vi "Add Marker.vi"(0 ".NET Refnum In":refnum<k24>, 1 "Inputs":T3, 3 "ToolTip Text":string="Base", 4 "Marker Tooltip":i32(ring) items=["On Mouse Over", "Never", "Always"], 5 "Marker Type":T1(ring)=enum."arrow") -> (8 "arrOverlayRefs":refnum<k24>[](array[refnum]), 12 ".NET Refnum Out":refnum<k24>, 14 "RefPointsColl - Out":refnum<k24>, 15 "arrPtKyOrId":string[](array[string]), 16 "arrLat|LngActv":dbl[][](array[numeric]), 17 "MarkersCount":i32, 18 "QFNs":cluster{"FN":T4, "Data":variant}[](array[cluster]))   [LabVIEW 2021, in "NMEA_GPS Ublox M8N.lvlib"]
uses:
  NMEA_GPS Ublox M8N.lvlib
  D:/My Projects/Ava Sanjesh Project/VI/GPS uBlox M8N Read/With GMap1.7.0/Data/GMap.NET.WindowsForms.dll
  Data/GMap.NET.WindowsForms.dll
  ctlSeqFNs.ctl
  ctlInput4PtsColl.ctl
  D:/My Projects/Ava Sanjesh Project/VI/GPS uBlox M8N Read/With GMap1.7.0/Data/GMap.NET.Core.dll
  Data/GMap.NET.Core.dll
  System.Drawing
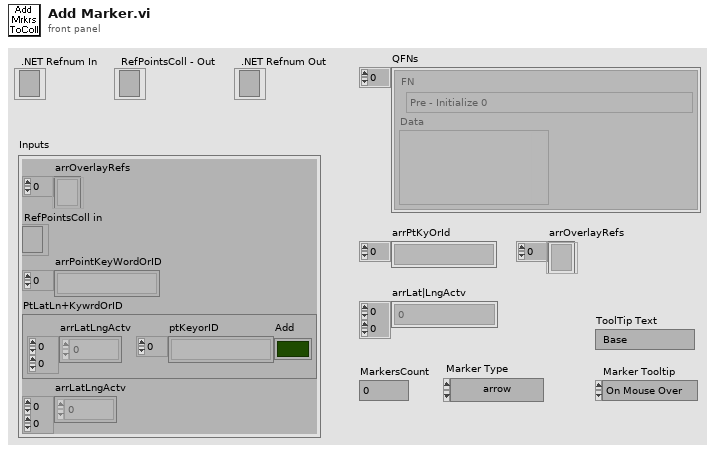
[diagram p1: front panel]
types:
  T1 = enum16{"none", "arrow", "blue", "blue_small", "blue_dot", "blue_pushpin", "brown_small", "gray_small", "green", "green_small", "green_dot", "green_pushpin", "green_big_go", "yellow", "yellow_small", "yellow_dot", "yellow_big_pause", "yellow_pushpin", "lightblue", "lightblue_dot", "lightblue_pushpin", "orange", "orange_small", "orange_dot", "pink", "pink_dot", "pink_pushpin", "purple", "purple_small", "purple_dot", "purple_pushpin", "red", "red_small", "red_dot", "red_pushpin", "red_big_stop", "black_small", "white_small"}
  T2 = typedef "NMEA_GPS Ublox M8N.lvlib/ctlInput4PtsColl.ctl" = cluster{"arrLatLngActv":dbl[][], "ptKeyorID":string[], "Add":bool}
  T3 = cluster{"arrOverlayRefs":refnum<k24>[], "RefPointsColl in":refnum<k24>, "arrPointKeyWordOrID":string[], "PtLatLn+KywrdOrID":T2, "arrLatLngActv":dbl[][]}
  T4 = typedef "NMEA_GPS Ublox M8N.lvlib/ctlSeqFNs.ctl" = enum16{"Pre - Initialize 0", "Pre - Initialize 1", "Pre - Initialize 2", "Pre - Initialize 3", "Idle", "Set Provider", "Set Scale", "Add Overlay", "Points - Create List (Container)", "Map - Marker Add Or Rmv", "Map - Markers Autofit", "Map - Markers Clear", "Error", "Exit"}
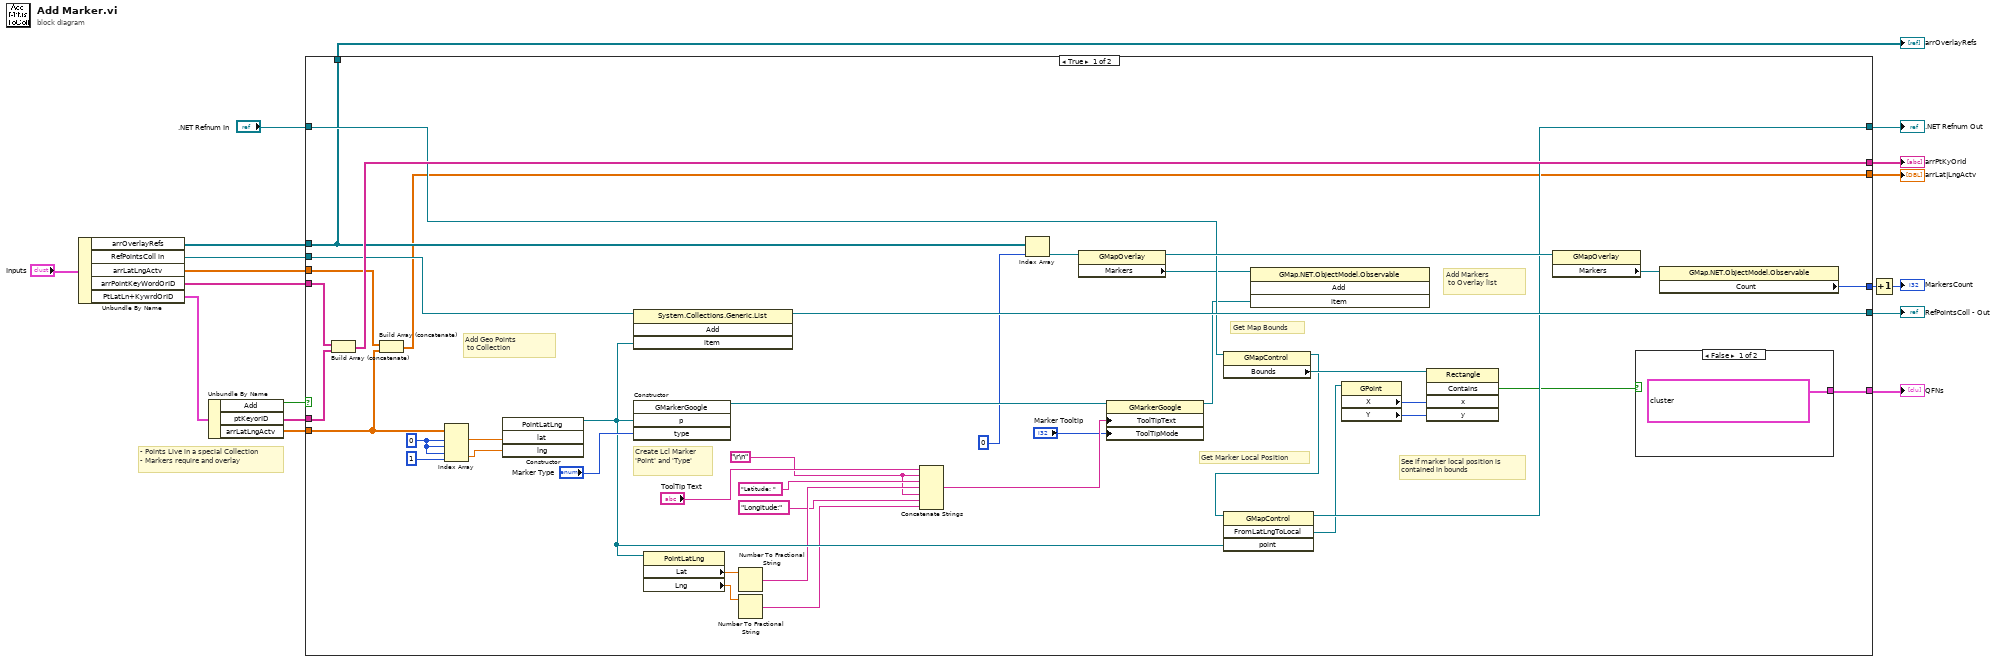
[diagram p0: block diagram]
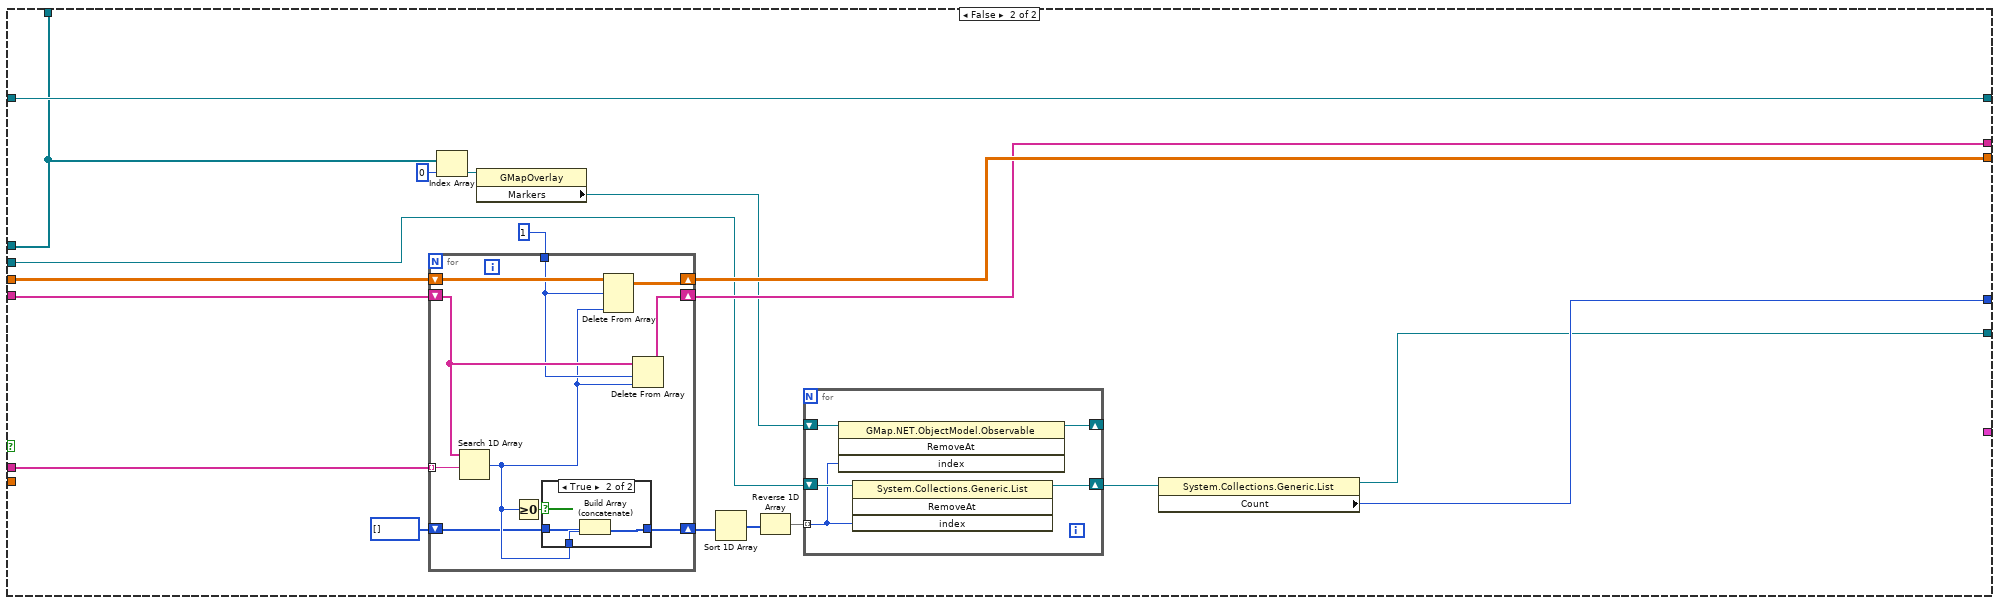
[diagram p3: hidden frame]
diagram:
  # "- Points Live in a special Collection\n- Markers require and overlay"
  n1 = Unbundle By Name("Inputs") -> ("arrOverlayRefs"=w10:refnum<k24>[], "RefPointsColl in"=w9:refnum<k24>, "arrLatLngActv"=w8:dbl[][], "arrPointKeyWordOrID"=w6:string[], "PtLatLn+KywrdOrID"=w7:T2)
  n2 = Unbundle By Name(w7) -> ("Add"=w2:bool, "ptKeyorID"=w12:string[], "arrLatLngActv"=w13:dbl[][])
  n3 = case shown="True" w2 {
    tunnel: [w60 _] -> w18
    tunnel: [w59 w74] -> w17
    tunnel: [w55 w75] -> w16
    tunnel: [w20 w76] -> w15
    tunnel: [w54 w65] -> w14
    tunnel: w13 -> [w53 _]
    tunnel: w12 -> [w52 w79]
    tunnel: w10 -> [w47 w63]
    tunnel: w9 -> [w51 w67]
    tunnel: w8 -> [w50 w78]
    tunnel: w6 -> [w49 w80]
    tunnel: ".NET Refnum In" -> [w48 w64]
    tunnel: [w46 w64] -> w3
    tunnel: [w47 w63] -> w4
    frame True {
      w25 = 0 ("index (row)")
      w29 = "\r\n"
      # "See if marker local position is \ncontained in bounds"
      # "Get Marker Local Position"
      # "Get Map Bounds"
      # "Add Markers\n to Overlay list"
      # "Create Lcl Marker  'Point' and 'Type'"
      # "Add Geo Points\n to Collection"
      n4 = Build Array (concatenate)(w49, w52) -> (w55:string[])
      n5 = Build Array (concatenate)(w50, w53) -> (w20:dbl[][])
      n6 = Index Array(array=w53, index (row) #1=w25, index (col) #1=w25, index (row) #2=w25, index (col) #2=1 ("disabled index (col)")) -> (element #1=w44:dbl, element #2=w43:dbl)
      n7 = constructor class="PointLatLng"("lat"=w44, "lng"=w43) -> (reference out=w33:refnum<k24>)  [unwired: 3 in, 4 out]
      n8 = invoke class="System.Collections.Generic.List" method="Add"(reference=w51, "item"=w33) -> (reference out=w54:refnum<k24>)  [unwired: 2 in, 3 out]
      n9 = constructor class="GMarkerGoogle"("p"=w33, "type"="Marker Type") -> (reference out=w41:refnum<k24>)  [unwired: 3 in, 4 out]
      n10 = property class="PointLatLng"(reference=w33) -> ("Lat"=w35:dbl, "Lng"=w34:dbl)  [unwired: 1 in, 2 out]
      n11 = Number To Fractional String(number=w35) -> (F-format string=w30:string)  [unwired: 3 in]
      n12 = Number To Fractional String(number=w34) -> (F-format string=w27:string)  [unwired: 3 in]
      n13 = Concatenate Strings("ToolTip Text", w29, "Latitude: " ("ToolTipText"), w30, w29, "Longitude:" ("ToolTipText"), w27) -> (w32:string)
      n14 = Index Array(array=w47, index=0) -> (element=w56:refnum<k24>)
      n15 = property class="GMapOverlay"(reference=w56) -> (reference out=w57:refnum<k24>, "Markers"=w22:refnum<k24>)  [unwired: 1 in, 1 out]
      n16 = property class="GMarkerGoogle"(reference=w41, "ToolTipText"=w32, "ToolTipMode"="Marker Tooltip") -> (reference out=w21:refnum<k24>)  [unwired: 1 in, 1 out]
      n17 = property class="GMapControl"(reference=w48) -> (reference out=w37:refnum<k24>, "Bounds"=w42:refnum<k24>)  [unwired: 1 in, 1 out]
      n18 = invoke class="GMapControl" method="FromLatLngToLocal"(reference=w37, "point"=w33) -> (reference out=w46:refnum<k24>, "FromLatLngToLocal"=w40:refnum<k24>)  [unwired: 2 in, 2 out]
      n19 = invoke class="GMap.NET.ObjectModel.Observable" method="Add"(reference=w22, "item"=w21) -> ()  [unwired: 2 in, 4 out]
      n20 = property class="GPoint"(reference=w40) -> ("X"=w39:i64, "Y"=w38:i64)  [unwired: 1 in, 2 out]
      n21 = invoke class="Rectangle" method="Contains"(reference=w42, "x"=w39, "y"=w38) -> ("Contains"=w23:bool)  [unwired: 2 in, 4 out]
      n22 = property class="GMapOverlay"(reference=w57) -> ("Markers"=w58:refnum<k24>)  [unwired: 1 in, 2 out]
      n23 = case shown="False" w23 {
        tunnel: [cluster{"Functions":T4, "Data":variant}[] [{"Functions"=enum."Map - Markers Autofit", "Data"=variant}, {"Functions"=enum."Set Scale", "Data"=variant}] ("QFNs") _] -> w60
        frame False {
        }
        frame True {
        }
      }
      n24 = property class="GMap.NET.ObjectModel.Observable"(reference=w58) -> ("Count"=w59:i32)  [unwired: 1 in, 2 out]
    }
    frame False {
      n25 = for {
        shift-right: [w91] -> w75
        shift-left: w80 -> [w93]
        tunnel: w79 -> [w95] mode=indexing
        shift-right: [w90] -> w76
        shift-left: w78 -> [w94]
        tunnel: 1 -> [w92]
        shift-right: [w87] -> w71
        shift-left: i32[] [] -> [w86]
        n26 = Search 1D Array(1D array=w93, element=w95) -> (index of element=w88:i32)  [unwired: 1 in]
        n27 = Greater Or Equal To 0?(x=w88) -> (x >= 0?=w89:bool)
        n28 = case shown="True" w89 {
          tunnel: w88 -> [_ w99]
          tunnel: [w96 w98] -> w87
          tunnel: w86 -> [w96 w97]
          frame False {
          }
          frame True {
            n29 = Build Array (concatenate)(w97, w99) -> (w98:i32[])
          }
        }
        n30 = Delete From Array(array=w94, length=w92, index (col)=w88) -> (array with subset deleted=w90:dbl[][])  [unwired: 1 in, 1 out]
        n31 = Delete From Array(array=w93, length=w92, index=w88) -> (array with subset deleted=w91:string[])  [unwired: 1 out]
      }
      n32 = Index Array(array=w63, index=0) -> (element=w73:refnum<k24>)
      n33 = property class="GMapOverlay"(reference=w73) -> ("Markers"=w68:refnum<k24>)  [unwired: 1 in, 2 out]
      n34 = Sort 1D Array(array=w71) -> (sorted array=w70:i32[])
      n35 = Reverse 1D Array(array=w70) -> (reversed array=w69:i32[])
      n36 = for {
        shift-right: [w84] -> w66
        shift-left: w67 -> [w85]
        shift-right: [w82] -> _
        shift-left: w68 -> [w83]
        tunnel: w69 -> [w81] mode=indexing
        n37 = invoke class="GMap.NET.ObjectModel.Observable" method="RemoveAt"(reference=w83, "index"=w81) -> (reference out=w82:refnum<k24>)  [unwired: 2 in, 3 out]
        n38 = invoke class="System.Collections.Generic.List" method="RemoveAt"(reference=w85, "index"=w81) -> (reference out=w84:refnum<k24>)  [unwired: 2 in, 3 out]
      }
      n39 = property class="System.Collections.Generic.List"(reference=w66) -> (reference out=w65:refnum<k24>, "Count"=w74:i32)  [unwired: 1 in, 1 out]
    }
  }
  "QFNs" <- w18
  "arrPtKyOrId" <- w16
  "arrLat|LngActv" <- w15
  "RefPointsColl - Out" <- w14
  "arrOverlayRefs" <- w4
  ".NET Refnum Out" <- w3
  n40 = Increment(x=w17) -> (x+1=→"MarkersCount":i32)
